vi "Profiler core.vi"(0 "Step number in":i32, 11 "error in":errorcluster) -> (4 "Step number out":i32, 15 "error out":errorcluster)   [LabVIEW 2014]
uses:
  <vilib>/Automated Test Systems Ltd/General Tools/Que lib/Read.vi
  <vilib>/Automated Test Systems Ltd/General Tools/Que lib/Que lib.lvlib
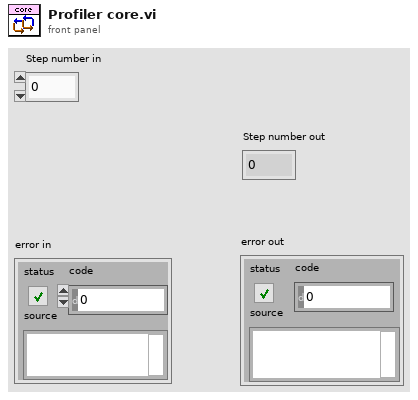
[diagram p1: front panel]
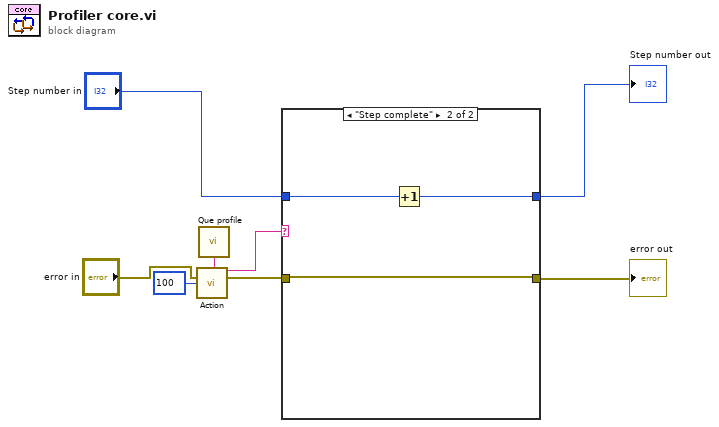
[diagram p0: block diagram]
diagram:
  n1 = call <vilib>:"Que profile.vi"() -> ("Que name"=w2:string)  [unwired: 15 in]
  n2 = call-poly <vilib>:"Action.vi"("Que name"=w2, "error in"="error in", "Timeout (default 2s)"=100) -> ("Message out"=w1:string, "error out"=w5:errorcluster)  [unwired: 10 in, 1 out]
  n3 = case shown="\"Step complete\"" w1 {
    tunnel: "Step number in" -> [w10 w13]
    tunnel: [w10 w12] -> w7
    tunnel: w5 -> [w9 w11]
    tunnel: [w9 w11] -> w6
    frame "False", Default {
    }
    frame "Step complete" {
      n4 = Increment(x=w13) -> (x+1=w12:i32)
    }
  }
  "Step number out" <- w7
  "error out" <- w6
